vi "Get Result for Target Blinks.vi"(10 "Target Blinks":u64, 11 "num":u64) -> (3 "Count":i32)   [LabVIEW 2024]
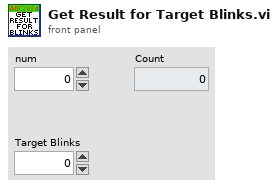
[diagram p1: front panel]
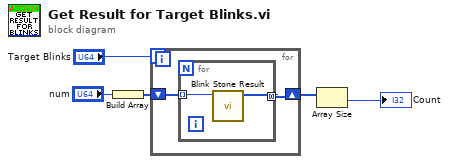
[diagram p0: block diagram]
diagram:
  n1 = Build Array("num") -> (w3:u64[])
  n2 = for {
    N: "Target Blinks" -> [_]
    shift-right: [w7] -> w4
    shift-left: w3 -> [w6]
    n3 = for {
      tunnel: w6 -> [w9] mode=indexing
      tunnel: [w8] -> w7 mode=concatenating
      n4 = call "Blink Stone Result.vi"("String"=w9) -> ("Result Array"=w8:u64[])  [unwired: 9 in, 1 out]
    }
  }
  n5 = Array Size(array=w4) -> (size(s)=→"Count":i32)
